vi "Get Tag Content.vi"(10 "Tag":string, 11 "xml string in":string) -> (1 "Type":string, 2 "Tag content":string, 3 "After end of tag":string)   [LabVIEW 2020, in "Advanced Assertions.lvlib"]
uses:
  Advanced Assertions.lvlib
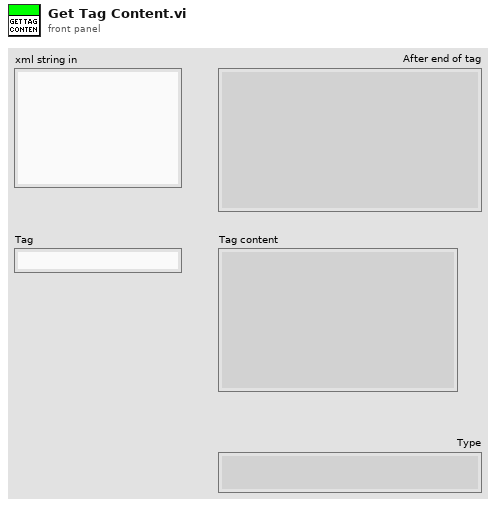
[diagram p1: front panel]
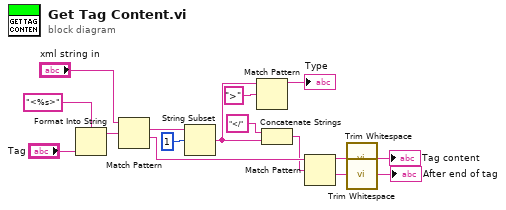
[diagram p0: block diagram]
diagram:
  n1 = Format Into String(format string="<%s>", "Tag") -> (resulting string=w16:string)  [unwired: 2 in, 1 out]
  n2 = Match Pattern(string="xml string in", regular expression=w16) -> (match substring=w5:string, after substring=w13:string)  [unwired: 1 in, 2 out]
  n3 = String Subset(string=w5, offset (0)=1) -> (substring=w4:string)  [unwired: 1 in]
  n4 = Match Pattern(string=w4, regular expression=">") -> (before substring=→"Type":string)  [unwired: 1 in, 3 out]
  n5 = Concatenate Strings("</" ("substring (\"\")"), w4) -> (w10:string)
  n6 = Match Pattern(string=w13, regular expression=w10) -> (before substring=w14:string, after substring=w11:string)  [unwired: 1 in, 2 out]
  n7 = call <vilib>:"Trim Whitespace.vi"("string"=w14) -> ("trimmed string"=→"Tag content":string)  [unwired: 1 in]
  n8 = call <vilib>:"Trim Whitespace.vi"("string"=w11) -> ("trimmed string"=→"After end of tag":string)  [unwired: 1 in]
